vi "TSV_2_DSC.vi"(8 "error in (no error)":errorcluster, 10 "Write to DSC?":bool, 11 "path to txt file":path) -> (0 "error out":errorcluster)   [LabVIEW 2016, in "VCL_2_DSC.lvclass"]
uses:
  VCL_2_DSC.lvclass
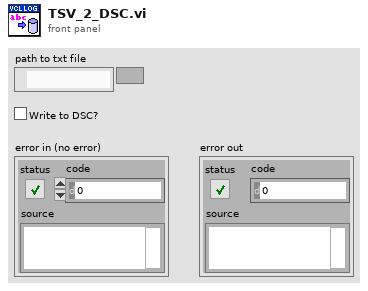
[diagram p1: front panel]
types:
  T1 = typedef "VCL_2_DSC.lvclass/TSLtoLV-cluster.ctl" = cluster{"time name":string, "trace name":string, "time array":timestamp[], "trace array":dbl[]}
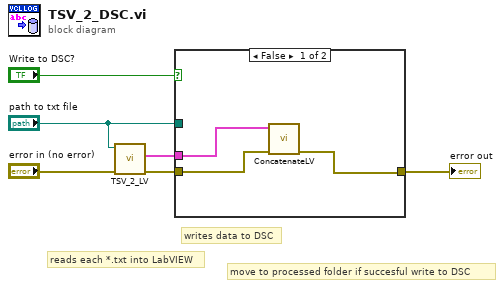
[diagram p0: block diagram]
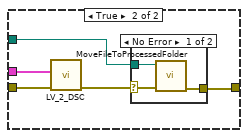
[diagram p2: hidden frame]
diagram:
  # "move to processed folder if succesful write to DSC"
  # "reads each *.txt into LabVIEW"
  # "writes data to DSC"
  n1 = call "TSV_2_LV.vi"("error in (no error)"="error in (no error)", "tsv file path (dialog if empty)"="path to txt file") -> ("error out"=w2:errorcluster, "data"=w3:T1[])  [unwired: 8 in]
  n2 = case shown="False" "Write to DSC?" {
    tunnel: w2 -> [w8 w14]
    tunnel: w3 -> [w9 w10]
    tunnel: [w7 w13] -> w4
    tunnel: "path to txt file" -> [_ w12]
    frame False {
      n3 = call "ConcatenateLV.vi"("error in (no error)"=w8, "data"=w9) -> ("error out"=w7:errorcluster)  [unwired: 9 in]
    }
    frame True {
      n4 = call "LV_2_DSC.vi"("error in (no error)"=w14, "data"=w10) -> ("error out"=w11:errorcluster)  [unwired: 9 in]
      n5 = case shown="No Error" w11 {
        selector: w11 -> [w15 w18]
        tunnel: [w17 w18] -> w13
        tunnel: w12 -> [w16 _]
        frame No Error {
          n6 = call "MoveFileToProcessedFolder.vi"("error in (no error)"=w15, "source file"=w16) -> ("error out"=w17:errorcluster)  [unwired: 8 in, 1 out]
        }
        frame Error {
        }
      }
    }
  }
  "error out" <- w4
